vi "2-6-2.vi"() -> ()   [LabVIEW 2022 SP3]
uses:
  2-6-3.vi
panel:
  out "布尔":bool
  out "仪表":dbl(knob) scale=0.0..10.0
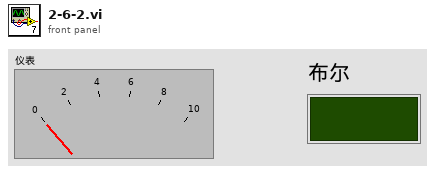
[diagram p1: front panel]
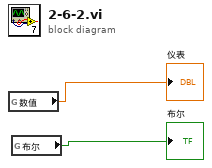
[diagram p0: block diagram]
diagram:
  n1 = global read "2-6-3.vi" "数值"() -> (→"仪表":dbl)
  n2 = global read "2-6-3.vi" "布尔"() -> (→"布尔":bool)
